vi "Additional_Post_Process_SJ_Data.vi"() -> ()   [LabVIEW 2012]
uses:
  Process_States.ctl
  Controls/SJ_Test_Matrix.ctl
  Controls/Analysis_info_cluster.ctl
  Controls/Inst_type.ctl
  Controls/Instrument_Array.ctl
  <vilib>/gmath/NumericalOptimization/stopping criteria.ctl
  <vilib>/gmath/NI_Gmath.lvlib
panel:
  out "New Filename":path=path "F:/Enflo_Data_Local/2011/Aero_Tunnel/nick_martin/Results_Post_Processed/11-2011/New_SJ_TestT_xls.dat"
  out "Prog bar":sgl(slide)=0.049707603 scale=0.0..1.0
  out "Message":string="Fitting parabolas to the data..."
  in  "Max Iterations":i32=3000
  in  "Tolerance":dbl=1e-06
  in  "Raw Data Folder":path=path "F:/Enflo_Data_Local/2011/Aero_Tunnel/nick_martin/Raw_Measurements/11-2011/New_SJ_TestT_xls"
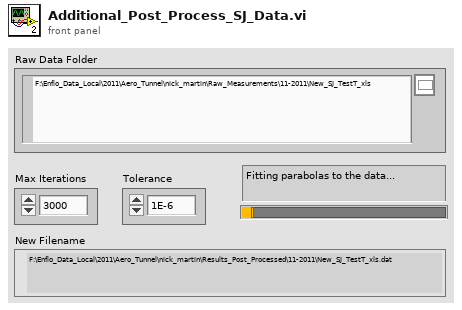
[diagram p1: front panel]
types:
  T1 = typedef "Process_States.ctl" = enum16{"Load Data", "Measured Calculations", "Fit Parabolas", "Save Data"}
  T2 = typedef "SJ_Test_Matrix.ctl" = cluster{"Channel Data":cluster{"Amplitude (V)":dbl, "Phase Average":dbl[][], "Phase Angle":dbl[], "Frequency (Hz)":dbl, "AS Freq":dbl, "Zero":dbl, "Analysis info cluster":T3, "Radius":dbl[], "||beta||":dbl, "Phi":dbl, "||xd'||":dbl, "xd":dbl[], "||xd||":dbl, "xd'":dbl[], "beta":dbl[]}[]}
  T3 = typedef "Analysis_info_cluster.ctl" = cluster{"Colour":u32, "Inst type":T4, "Inst name":string, "Symbol":string, "Code name":string, "Extra Info":string, "Inst Array":T5, "Extra Titles":string[], "Extra Values":string[], "U":dbl, "u^2":dbl, "u^3":dbl, "u^4":dbl, "Skew_u":dbl, "Kurt_u":dbl, "Sd Error in Mean":dbl, "% u'/U":dbl, "X":dbl, "Y":dbl, "Z":dbl, "Timescale integral to 25%":dbl, "Sd Error in Variance":dbl, "Calib File":path, "Calib Constants":dbl[], "Output Position":bool, "Full Stats":bool, "Av Sampling Rate":dbl, "Av No of Samples":dbl, "Total Meas Time (s)":dbl, "ADAM Ch Name":string}
  T4 = typedef "Inst_type.ctl" = enum16{"Propeller anemometer", "Raw voltage", "Pressure Transducer", "Pitot-static tube", "Preston tube", "Hot wire", "Cross wire 1", "Cross wire 2", "Generic Linear", "Generic Polynomial", "Generic BackPoly", "Fast FID", "Thermocouple", "Cold wire", "Pulsed Wire", "LDA Vel", "LDA Tran time", "LDA Arr time"}
  T5 = typedef "Instrument_Array.ctl" = enum16{"PWA", "LDA", "Analogue"}
  T6 = typedef "NI_Gmath.lvlib/stopping criteria.ctl" = cluster{"function tolerance":dbl, "parameter tolerance":dbl, "max iterations":i32, "max function calls":i32, "gradient tolerance":dbl, "max time (sec)":dbl}
  T7 = cluster{"Amplitude (V)":dbl, "Phase Average":dbl[][], "Phase Angle":dbl[], "Frequency (Hz)":dbl, "AS Freq":dbl, "Zero":dbl, "Analysis info cluster":T3, "Radius":dbl[], "||beta||":dbl, "Phi":dbl, "||xd'||":dbl, "xd":dbl[], "||xd||":dbl, "xd'":dbl[], "beta":dbl[]}[]
  T8 = cluster{"Amplitude (V)":dbl, "Phase Average":dbl[][], "Phase Angle":dbl[], "Frequency (Hz)":dbl, "AS Freq":dbl, "Zero":dbl, "Analysis info cluster":T3, "Radius":dbl[], "||beta||":dbl, "Phi":dbl, "||xd'||":dbl, "xd":dbl[], "||xd||":dbl, "xd'":dbl[], "beta":dbl[]}
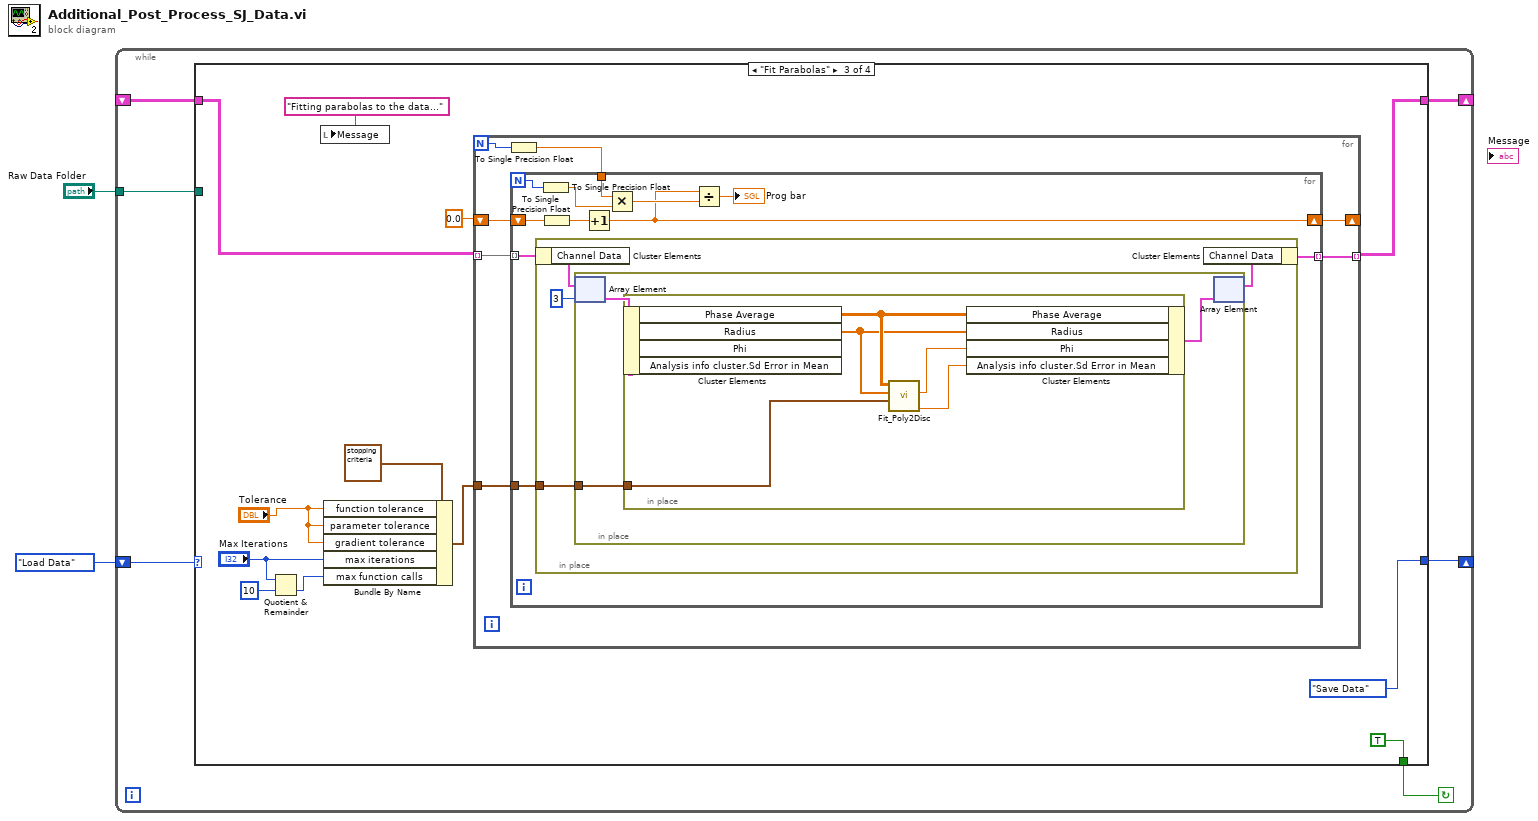
[diagram p0: block diagram]
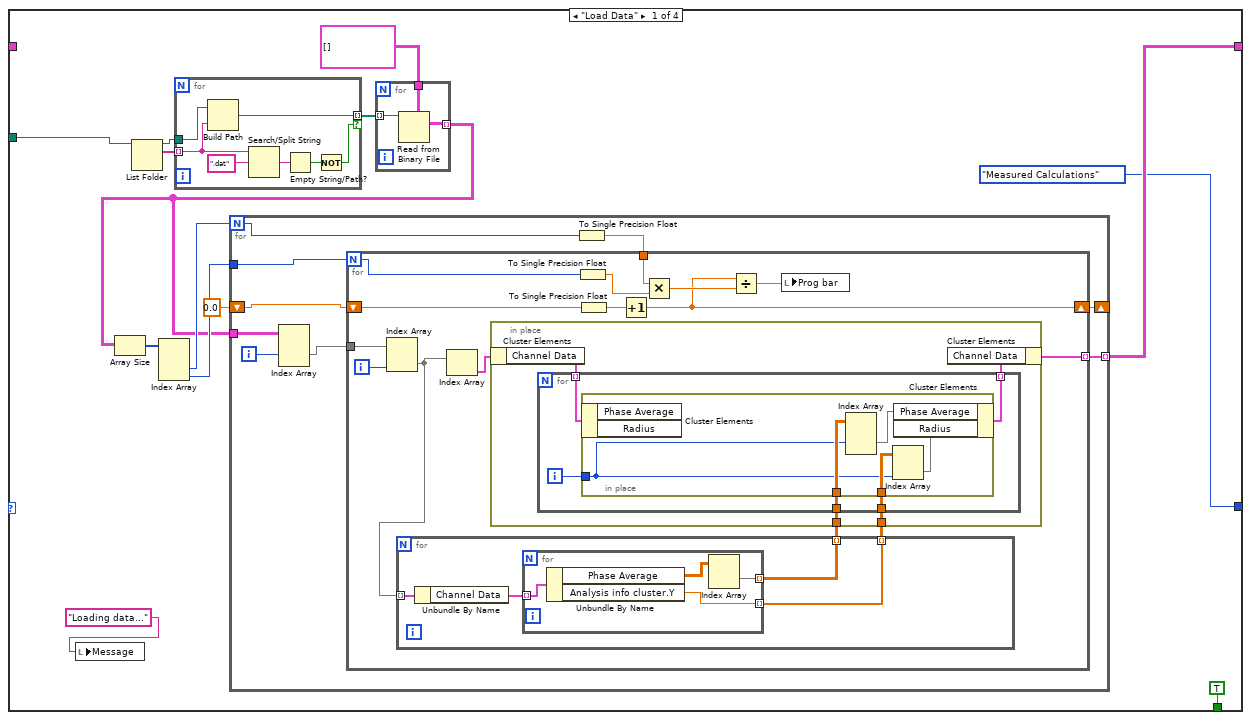
[diagram p2: hidden frame]
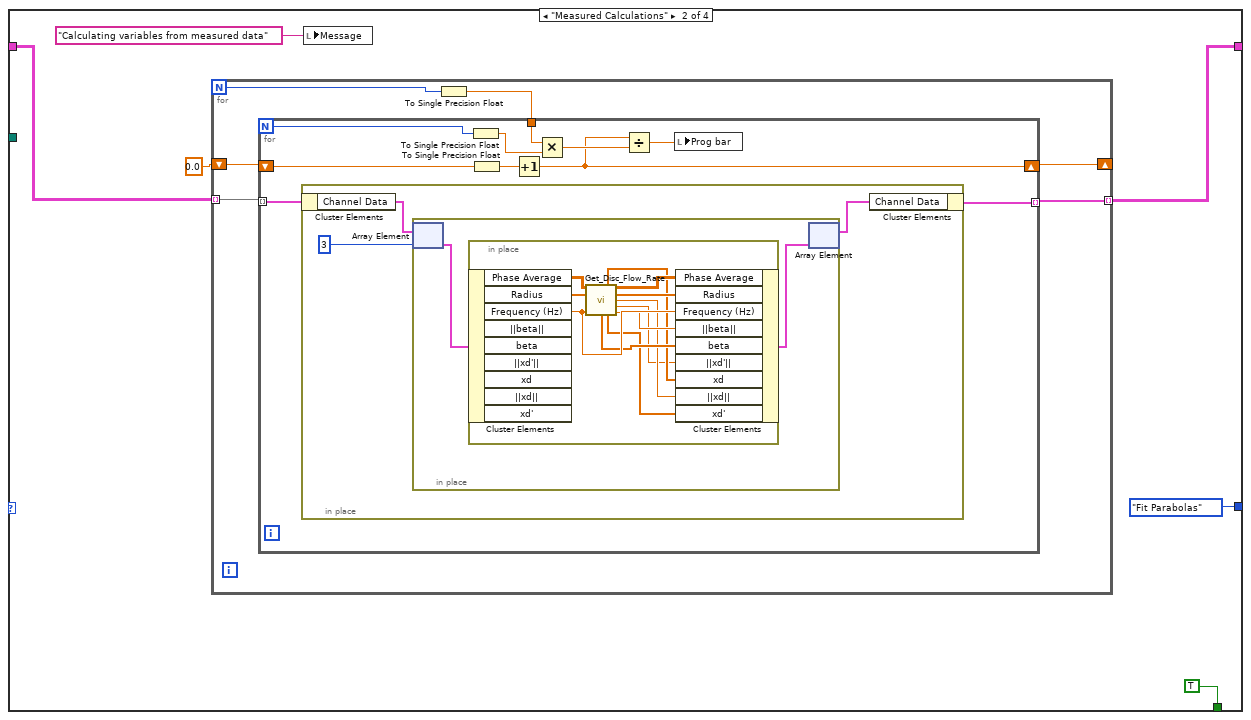
[diagram p3: hidden frame]
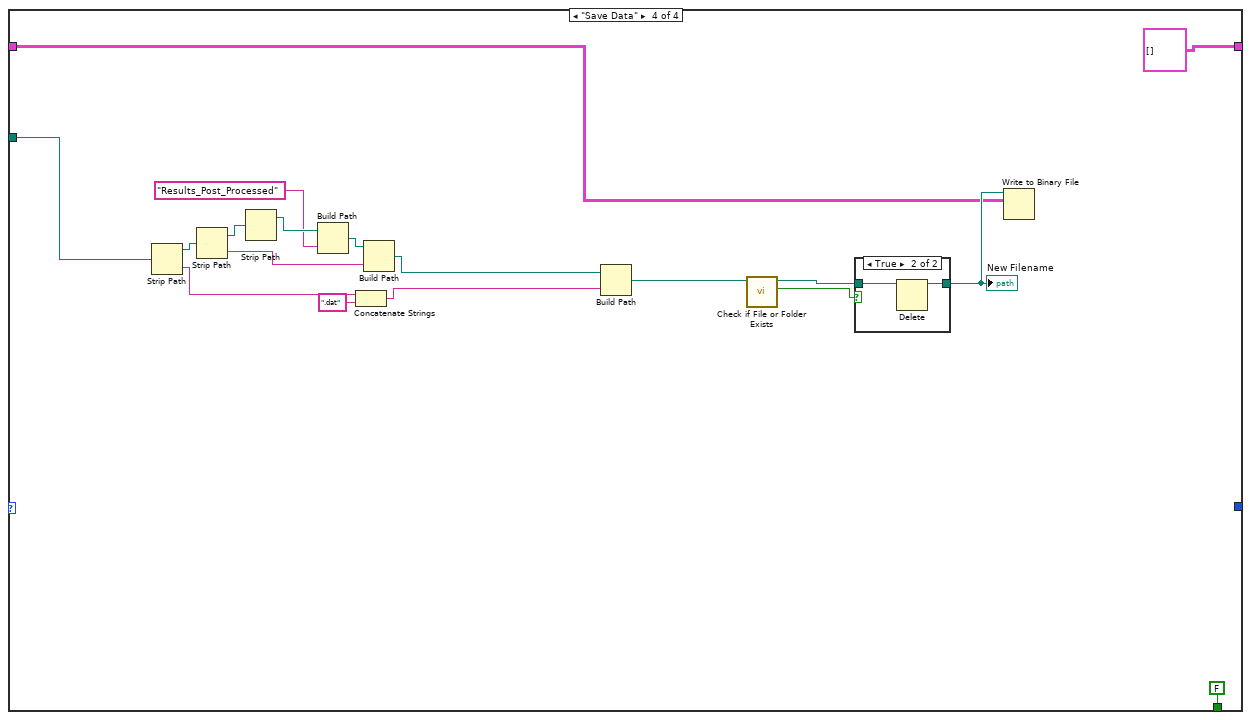
[diagram p4: hidden frame]
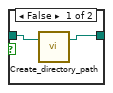
[diagram p5: hidden frame]
diagram:
  n1 = while {
    shift-right: [w7] -> _
    shift-left: _ -> [w6]
    shift-right: [w5] -> _
    shift-left: Process_States."Load Data" -> [w8]
    tunnel: "Raw Data Folder" -> [w3]
    stop <- w4 continue-if-true
    n2 = case shown="\"Fit Parabolas\"" w8 {
      tunnel: [w19 w81 w119 T2[][] []] -> w7
      tunnel: w6 -> [_ w82 w120 w159]
      tunnel: [Process_States."Measured Calculations" ("Enum") Process_States."Fit Parabolas" ("Enum") Process_States."Save Data" ("Enum") _] -> w5
      tunnel: [TRUE TRUE TRUE FALSE] -> w4
      tunnel: w3 -> [w11 _ _ w163]
      frame "Load Data" {
        n3 = local write "Message"("Loading data..." ("Message")) -> ()
        n4 = List Folder(path=w11) -> (path out=w14:path, filenames=w13:string[])  [unwired: 3 in, 2 out]
        n5 = for {
          tunnel: w13 -> [w27] mode=indexing
          tunnel: [w26] -> w15 mode=indexing if=w30
          tunnel: w14 -> [w28]
          n6 = Build Path(base path=w28, name or relative path=w27) -> (appended path=w26:path)
          n7 = Search/Split String(string=w27, search string/char (-)=".dat" ("regular expression")) -> (match + rest of string=w29:string)  [unwired: 1 in, 2 out]
          n8 = Empty String/Path?(string/path=w29) -> (empty?=w31:bool)
          n9 = Not(x=w31) -> (.not. x?=w30:bool)
        }
        n10 = for {
          tunnel: w15 -> [w25] mode=indexing
          tunnel: T2[][] [] -> [w24]
          tunnel: [w23] -> w12 mode=indexing
          n11 = Read from Binary File(5:w24, 11:w25) -> (2:w23:T2[][])  [unwired: 4 in, 3 out]
        }
        n12 = Array Size(array=w12) -> (size(s)=w22:i32[])
        n13 = Index Array(array=w22) -> (element #2=w21:i32, element #3=w20:i32)  [unwired: 3 in, 1 out]
        n14 = for {
          N: w21 -> [w35]
          tunnel: w12 -> [w41]
          tunnel: w20 -> [w38]
          tunnel: [w37] -> w19 mode=indexing
          shift-right: [w34] -> _
          shift-left: sgl 0.0 -> [w33]
          i -> [w40]
          n15 = Index Array(array=w41, index (dim 1)=w40) -> (element=w39:T2[][])  [unwired: 2 in]
          n16 = To Single Precision Float(number=w35) -> (single precision float=w36:sgl)
          n17 = for {
            N: w38 -> [w44]
            tunnel: w39 -> [w56]
            tunnel: [w50] -> w37 mode=indexing
            tunnel: w36 -> [w45]
            shift-right: [w43] -> w34
            shift-left: w33 -> [w42]
            i -> [w55]
            n18 = Index Array(array=w56, index (col)=w55) -> (element=w54:T2[])  [unwired: 1 in]
            n19 = for {
              tunnel: w54 -> [w74] mode=indexing
              tunnel: [w71] -> w52 mode=indexing
              tunnel: [w72] -> w51 mode=indexing
              n20 = Unbundle By Name(w74) -> ("Channel Data"=w73:T7)
              n21 = for {
                tunnel: [w78] -> w72 mode=indexing
                tunnel: [w75] -> w71 mode=indexing
                tunnel: w73 -> [w76] mode=indexing
                n22 = Unbundle By Name(w76) -> ("Phase Average"=w77:dbl[][], "Analysis info cluster.Y"=w78:dbl)
                n23 = Index Array(array=w77) -> (element=w75:dbl[])  [unwired: 2 in]
              }
            }
            n24 = Index Array(array=w54) -> (element=w53:T2)  [unwired: 1 in]
            n25 = in-place {
              in-place-border: w52 -> [w60]
              in-place-border: w51 -> [w59]
              n26 = in-place-cluster #1(w53) -> ("Channel Data"=w57:T7)
              n27 = for {
                tunnel: w60 -> [w62]
                tunnel: w59 -> [w61]
                tunnel: [w65] -> w58 mode=indexing
                tunnel: w57 -> [w64] mode=indexing
                i -> [w63]
                n28 = in-place {
                  in-place-border: w62 -> [w70]
                  in-place-border: w63 -> [w67]
                  in-place-border: w61 -> [w68]
                  n29 = in-place-cluster #2(w64) -> ()  [unwired: 2 out]
                  n30 = Index Array(array=w70, index (dim 1)=w67) -> (element=w69:dbl[][])  [unwired: 2 in]
                  n31 = Index Array(array=w68, index (col)=w67) -> (element=w66:dbl[])  [unwired: 1 in]
                  n32 = in-place-cluster #2("Phase Average"=w69, "Radius"=w66) -> (w65:T8)
                }
              }
              n33 = in-place-cluster #1("Channel Data"=w58) -> (w50:T2)
            }
            n34 = To Single Precision Float(number=w44) -> (single precision float=w46:sgl)
            n35 = To Single Precision Float(number=w42) -> (single precision float=w48:sgl)
            n36 = Increment(x=w48) -> (x+1=w43:sgl)
            n37 = Multiply(x=w45, y=w46) -> (x*y=w47:sgl)
            n38 = Divide(x=w43, y=w47) -> (x/y=w49:sgl)
            n39 = local write "Prog bar"(w49) -> ()
          }
        }
      }
      frame "Measured Calculations" {
        n40 = for {
          N -> [w89]
          tunnel: w82 -> [w90] mode=indexing
          tunnel: [w88] -> w81 mode=indexing
          shift-right: [w85] -> _
          shift-left: sgl 0.0 ("single precision float") -> [w86]
          n41 = To Single Precision Float(number=w89) -> (single precision float=w87:sgl)
          n42 = for {
            N -> [w99]
            tunnel: w90 -> [w100] mode=indexing
            tunnel: w87 -> [w97]
            tunnel: [w95] -> w88 mode=indexing
            shift-right: [w92] -> w85
            shift-left: w86 -> [w94]
            n43 = in-place {
              n44 = in-place-cluster #3(w100) -> ("Channel Data"=w103:T7)
              n45 = in-place {
                n46 = in-place-array #4(w103, 3) -> (w105:T8)
                n47 = in-place {
                  n48 = in-place-cluster #5(w105) -> ("Phase Average"=w116:dbl[][], "Radius"=w115:dbl[], "Frequency (Hz)"=w114:dbl)  [unwired: 6 out]
                  n49 = call "Get_Disc_Flow_Rate.vi"("Phase Average (mm)"=w116, "Radius (mm)"=w115, "Jet Frequency"=w114) -> ("xd(t)"=w109:dbl[], "xd(t,r)"=w111:dbl[][], "Radius (m)"=w110:dbl[], "||xd||"=w108:dbl, "||xd'||"=w106:dbl, "beta"=w112:dbl[], "xd'(t)"=w107:dbl[], "||beta||"=w113:dbl)  [unwired: 4 in, 1 out]
                  n50 = in-place-cluster #5("Phase Average"=w111, "Radius"=w110, "Frequency (Hz)"=w114, "||beta||"=w113, "beta"=w112, "||xd'||"=w106, "xd"=w109, "||xd||"=w108, "xd'"=w107) -> (w104:T8)
                }
                n51 = in-place-array #4(w104) -> (w101:T7)  [unwired: 1 out]
              }
              n52 = in-place-cluster #3("Channel Data"=w101) -> (w95:T2)
            }
            n53 = To Single Precision Float(number=w99) -> (single precision float=w98:sgl)
            n54 = To Single Precision Float(number=w94) -> (single precision float=w93:sgl)
            n55 = Increment(x=w93) -> (x+1=w92:sgl)
            n56 = Multiply(x=w97, y=w98) -> (x*y=w96:sgl)
            n57 = Divide(x=w92, y=w96) -> (x/y=w91:sgl)
            n58 = local write "Prog bar"(w91) -> ()
          }
        }
        n59 = local write "Message"("Calculating variables from measured data" ("Message")) -> ()
      }
      frame "Fit Parabolas" {
        n60 = Quotient & Remainder(x="Max Iterations", y=10) -> (floor(x/y)=w122:i32)  [unwired: 1 out]
        n61 = local write "Message"("Fitting parabolas to the data..." ("Message")) -> ()
        n62 = Bundle By Name(cluster=T6 {"function tolerance"=0.001, "parameter tolerance"=0.001, "max iterations"=100, "max function calls"=1000, "gradient tolerance"=0.001, "max time (sec)"=-1.0} ("stopping criteria"), "function tolerance"="Tolerance", "parameter tolerance"="Tolerance", "gradient tolerance"="Tolerance", "max iterations"="Max Iterations", "max function calls"=w122) -> (w125:T6)
        n63 = for {
          N -> [w133]
          tunnel: w120 -> [w135] mode=indexing
          tunnel: w125 -> [w134]
          tunnel: [w132] -> w119 mode=indexing
          shift-right: [w129] -> _
          shift-left: sgl 0.0 ("single precision float") -> [w130]
          n64 = To Single Precision Float(number=w133) -> (single precision float=w131:sgl)
          n65 = for {
            N -> [w144]
            tunnel: w135 -> [w146] mode=indexing
            tunnel: w134 -> [w145]
            tunnel: w131 -> [w142]
            tunnel: [w140] -> w132 mode=indexing
            shift-right: [w136] -> w129
            shift-left: w130 -> [w138]
            n66 = in-place {
              in-place-border: w145 -> [w147]
              n67 = in-place-cluster #6(w146) -> ("Channel Data"=w150:T7)
              n68 = in-place {
                in-place-border: w147 -> [w152]
                n69 = in-place-array #7(w150, 3) -> (w153:T8)
                n70 = in-place {
                  in-place-border: w152 -> [w158]
                  n71 = in-place-cluster #8(w153) -> ("Phase Average"=w157:dbl[][], "Radius"=w156:dbl[])  [unwired: 2 out]
                  n72 = call "Fit_Poly2Disc.vi"("stopping criteria"=w158, "Rc"=w156, "Xd(t,r)"=w157) -> ("f(minimum)"=w154:dbl, "Sine Phase"=w155:dbl)  [unwired: 6 in, 1 out]
                  n73 = in-place-cluster #8("Phase Average"=w157, "Radius"=w156, "Phi"=w155, "Analysis info cluster.Sd Error in Mean"=w154) -> (w151:T8)
                }
                n74 = in-place-array #7(w151) -> (w148:T7)  [unwired: 1 out]
              }
              n75 = in-place-cluster #6("Channel Data"=w148) -> (w140:T2)
            }
            n76 = To Single Precision Float(number=w144) -> (single precision float=w143:sgl)
            n77 = To Single Precision Float(number=w138) -> (single precision float=w137:sgl)
            n78 = Increment(x=w137) -> (x+1=w136:sgl)
            n79 = Multiply(x=w142, y=w143) -> (x*y=w141:sgl)
            n80 = Divide(x=w136, y=w141) -> (x/y=→"Prog bar":sgl)
          }
        }
      }
      frame "Save Data" {
        n81 = Strip Path(path=w163) -> (stripped path=w171:path, name=w162:string)
        n82 = Strip Path(path=w171) -> (stripped path=w170:path, name=w166:string)
        n83 = Strip Path(path=w170) -> (stripped path=w169:path)  [unwired: 1 out]
        n84 = Build Path(base path=w169, name or relative path="Results_Post_Processed") -> (appended path=w167:path)
        n85 = Concatenate Strings(w162, ".dat" ("string")) -> (w160:string)
        n86 = Build Path(base path=w167, name or relative path=w166) -> (appended path=w165:path)
        n87 = Build Path(base path=w165, name or relative path=w160) -> (appended path=w164:path)
        n88 = call <vilib>:"Check if File or Folder Exists.vi"("path"=w164) -> ("file or folder exists?"=w174:bool, "dup path"=w173:path)  [unwired: 8 in, 1 out]
        n89 = case shown="True" w174 {
          tunnel: w173 -> [w178 w180]
          tunnel: [w177 w179] -> w172
          frame False {
            n90 = call "Create_directory_path.vi"("Path name"=w178) -> ("Path name Out"=w177:path)  [unwired: 1 in, 1 out]
          }
          frame True {
            n91 = Delete(path (use dialog)=w180) -> (deleted path=w179:path)  [unwired: 4 in, 2 out]
          }
        }
        "New Filename" <- w172
        n92 = Write to Binary File(file (use dialog)=w172, data=w159) -> ()  [unwired: 4 in, 3 out]
      }
    }
  }
